vi "SystemMessageDialogBox_DynamicLaunch.vi"(6 "ErrorMessageToProcess":errorcluster, 8 "ErrorIn":errorcluster, 9 "Timeout (-1)":i32=-1, 10 "CorrAct":string, 11 "Source":string) -> (0 "ErrorOut":errorcluster)   [LabVIEW 2018]
doc: "Call this modal dialog when an error occurs. This VI logs the error to a file to aid in diagnosis.\n\nThe CorrAct (Corrective Action) input can be used to suggest a solution to the user.\n\nCopyright © 2016 Epimedia, Inc. All Rights Reserved.\n\nThe Epimedia Application Library is Copyright © 2009-2016 Epimedia, Inc. \nAll Rights Reserved. Used under license."
uses:
  Controls/SMSDataCluster.ctl
  <vilib>/Utility/sysdir.llb/System Directory Type.ctl
panel:
  in  "SMS":T1
  in  "Close":bool
  out "CorrAction":string caption="Corrective Action:"
  out "ErrorSource":string caption="Source:"
  out "ErrorCode":i32 caption="Code:"
  # "System Message"
  # "Copyright © 2016 Epimedia, Inc. All Rights Reserved.\n\nThe Epimedia Application Library is Copyright © 2009-2016 Epimedia, Inc. \nAll Rights Reserved. Used under license."
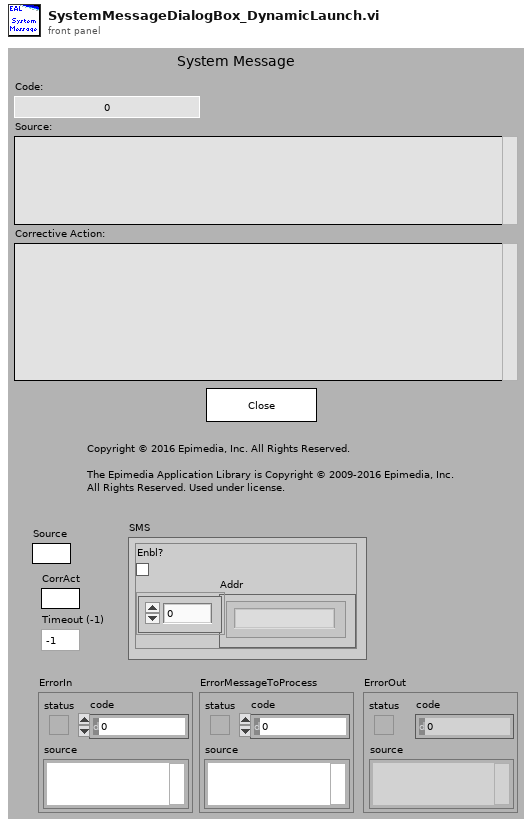
[diagram p1: front panel]
types:
  T1 = typedef "SMSDataCluster.ctl" = cluster{"Enbl?":bool, "Addr":string[]}
  T2 = enum8{"Enabled", "Disabled", "Disabled and Grayed Out"}
  T3 = typedef "System Directory Type.ctl" = i32
  T4 = enum16{"open", "replace", "create", "open or create", "replace or create", "replace or create with confirmation"}
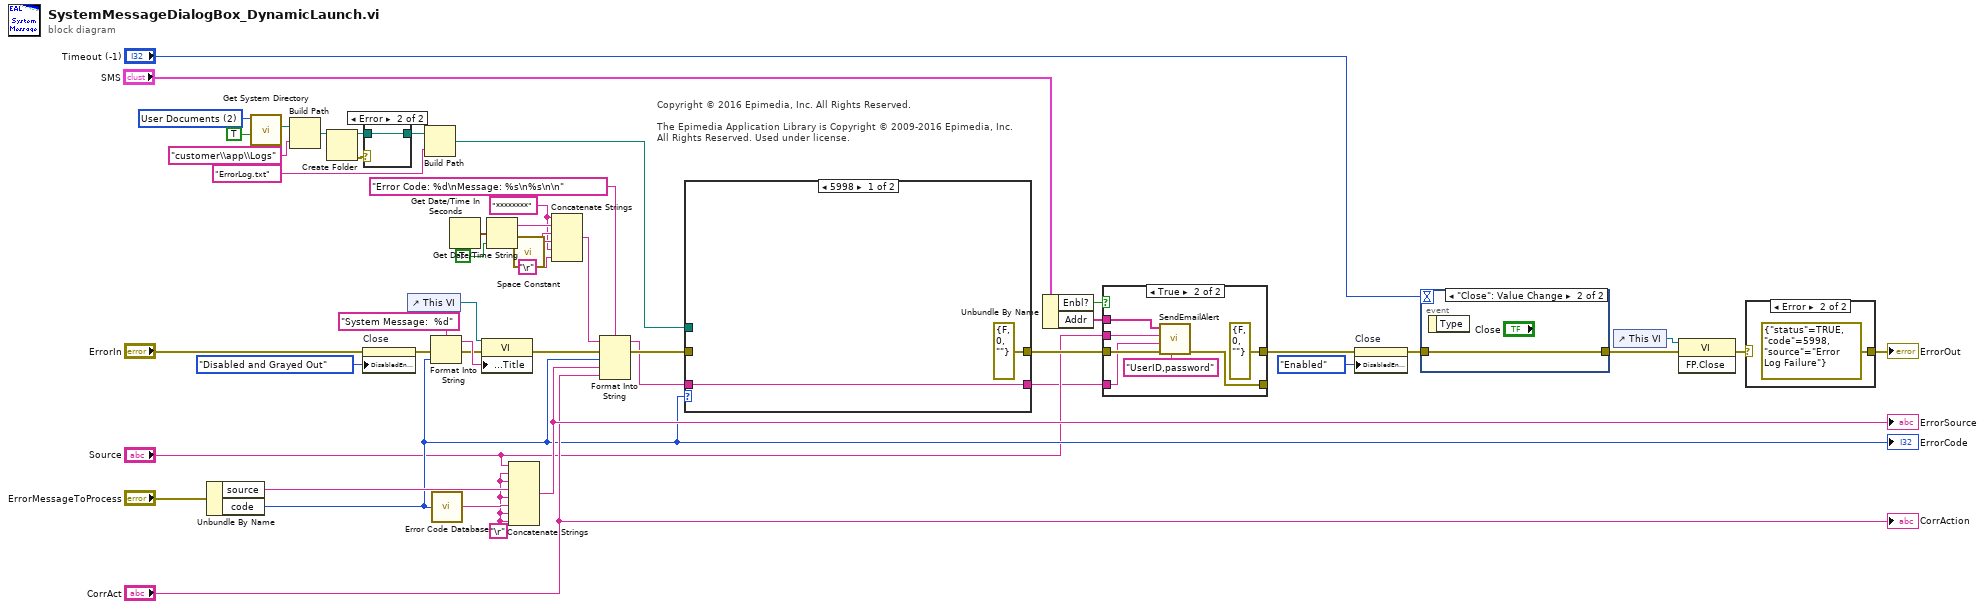
[diagram p0: block diagram]
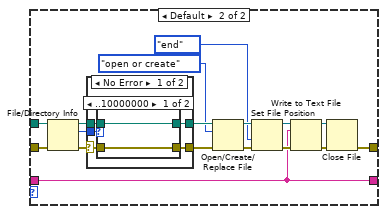
[diagram p3: hidden frame]
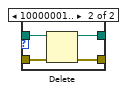
[diagram p4: hidden frame]
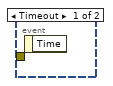
[diagram p8: hidden frame]
diagram:
  w38 = T3 2 items=["User Home"=0, "User Desktop"=1, "User Documents"=2, "User Application Data"=3, "User Preferences"=4, "User Temporary"=5, "Public Documents"=6, "Public Application Data"=7, "Public Preferences"=8, "Public Cache"=13, "System Core Libraries"=9, "System Installed Libraries"=10, "Application Files"=11, "Boot Volume Root"=12] ("system directory type")
  w41 = "********" ("string")
  w22 = "\r"
  # "Copyright © 2016 Epimedia, Inc. All Rights Reserved.\n\nThe Epimedia Application Library is Copyright © 2009-2016 Epimedia, Inc. \nAll Rights Reserved. Used under license."
  n1 = Unbundle By Name("ErrorMessageToProcess") -> ("source"=w23:string, "code"=w6:i32)
  "ErrorCode" <- w6
  n2 = call <vilib>:"Get System Directory.vi"("create directory if not found? (F)"=TRUE, "system directory type"=w38) -> ("system directory"=w37:path)  [unwired: 9 in]
  n3 = Build Path(base path=w37, name or relative path="customer\\app\\Logs") -> (appended path=w30:path)
  n4 = Create Folder(path (use dialog)=w30) -> (created path=w32:path, error out=w33:errorcluster)  [unwired: 2 in, 1 out]
  n5 = property on="Close" class="Bool"(error in="ErrorIn", "DisabledEnum"=T2."Disabled and Grayed Out" ("Disabled")) -> (error out=w20:errorcluster)  [unwired: 1 in, 1 out]
  n6 = case shown="Error" w33 {
    tunnel: w32 -> [w51 w52]
    tunnel: [w51 w52] -> w31
    frame No Error {
    }
    frame Error {
    }
  }
  n7 = control-ref of="This VI"() -> (w28:refnum<vi>)
  n8 = Build Path(base path=w31, name or relative path="ErrorLog.txt") -> (appended path=w29:path)
  n9 = Format Into String(format string="System Message:  %d" ("string"), error in=w20, w6) -> (resulting string=w26:string, error out=w25:errorcluster)  [unwired: 1 in]
  n10 = call <vilib>:"Error Code Database.vi"("Error Code"=w6) -> ("Error Text"=w42:string)
  n11 = Get Date/Time In Seconds() -> (seconds since 1Jan1904=w49:timestamp)
  n12 = property class="VI"(reference=w28, error in=w25, "Front Panel.Title"=w26) -> (error out=w24:errorcluster)  [unwired: 1 out]
  n13 = Get Date/Time String(seconds (now)=w49, want seconds? (F)=TRUE) -> (date string=w48:string, time string=w47:string)  [unwired: 1 out]
  n14 = Concatenate Strings("Source", w22, w22, w23, w22, w42, w22, w22) -> (w15:string)
  "ErrorSource" <- w15
  n15 = call <vilib>:"Space Constant.vi"() -> ("String"=w45:string)
  n16 = Concatenate Strings(w41, w48, w45, w47, w41, "\r") -> (w43:string)
  n17 = Format Into String(format string="Error Code: %d\nMessage: %s\n%s\n\n", initial string=w43, error in=w24, w6, w15, "CorrAct") -> (resulting string=w12:string, error out=w36:errorcluster)
  n18 = case shown="5998" w6 {
    tunnel: w36 -> [_ w58]
    tunnel: w29 -> [_ w57]
    tunnel: [errorcluster {"status"=FALSE, "code"=0, "source"=""} ("error out") w56] -> w7
    tunnel: w12 -> [w53 w55]
    tunnel: [w53 w55] -> w4
    frame 5998 {
    }
    frame Default {
      n19 = File/Directory Info(path=w57, error in=w58) -> (path out=w68:path, size=w70:i64, error out=w71:errorcluster)  [unwired: 4 out]
      n20 = case shown="No Error" w71 {
        selector: w71 -> [w72 _]
        tunnel: [w76 _] -> w67
        tunnel: w68 -> [w75 w83]
        tunnel: [w74 w83] -> w69
        tunnel: w70 -> [w73 _]
        frame No Error {
          n21 = case shown="..10000000" w73 {
            tunnel: w72 -> [w77 w82]
            tunnel: [w77 w81] -> w76
            tunnel: w75 -> [w78 w80]
            tunnel: [w78 w79] -> w74
            frame ..10000000 {
            }
            frame 10000001.. {
              n22 = Delete(path (use dialog)=w80, error in=w82) -> (deleted path=w79:path, error out=w81:errorcluster)  [unwired: 3 in, 1 out]
            }
          }
        }
        frame Error {
        }
      }
      n23 = Open/Create/Replace File(file path (use dialog)=w69, error in=w67, operation (0:open)=T4."open or create") -> (refnum out=w64:refnum<file>, error out=w63:errorcluster)  [unwired: 4 out]
      n24 = Set File Position(refnum=w64, from (0:start)=enum16{"start", "end", "current"}."end", error in=w63) -> (refnum out=w65:refnum<file>, error out=w66:errorcluster)  [unwired: 1 out]
      n25 = Write to Text File(file (use dialog)=w65, text=w55, error in=w66) -> (refnum out=w61:refnum<file>, error out=w60:errorcluster)  [unwired: 2 out]
      n26 = Close File(refnum=w61, error in=w60) -> (error out=w56:errorcluster)  [unwired: 1 out]
    }
  }
  n27 = Unbundle By Name("SMS") -> ("Enbl?"=w2:bool, "Addr"=w1:string[])
  n28 = case shown="True" w2 {
    tunnel: w7 -> [w84 w91]
    tunnel: [w84 errorcluster {"status"=FALSE, "code"=0, "source"=""} ("ErrorOut")] -> w8
    tunnel: [_ w89] -> _
    tunnel: "Source" -> [_ w87]
    tunnel: w4 -> [_ w86]
    tunnel: w1 -> [_ w85]
    frame False {
    }
    frame True {
      n29 = call "SendEmailAlert.vi"("UserID,PW"="UserID,password", "ErrorIn"=w91, "Body"=w86, "Subject"=w87, "RecipientsIn"=w85) -> ("ErrorOut"=w89:errorcluster)  [unwired: 6 in]
    }
  }
  n30 = property on="Close" class="Bool"(error in=w8, "DisabledEnum"=T2."Enabled" ("Disabled")) -> (error out=w17:errorcluster)  [unwired: 1 in, 1 out]
  n31 = event shown="[1] \"Close\": Value Change" {
    selector: _ -> [_ _]
    dyn-events: _ -> [_ _]
    timeout: "Timeout (-1)" -> [_ _]
    tunnel: w17 -> [_ w92]
    tunnel: [_ w92] -> w16
    event Timeout {
      n32 = event-data() -> ()  [unwired: 2 out]
    }
    event "Close": Value Change {
      n33 = event-data() -> ()  [unwired: 2 out]
    }
  }
  n34 = control-ref of="This VI"() -> (w11:refnum<vi>)
  n35 = invoke class="VI" method="FP.Close"(reference=w11, error in=w16) -> (error out=w10:errorcluster)  [unwired: 1 in, 2 out]
  n36 = case shown="Error" w10 {
    selector: w10 -> [w93 _]
    tunnel: [w93 errorcluster {"status"=TRUE, "code"=5998, "source"="Error Log Failure"} ("error IO")] -> w9
    frame No Error {
    }
    frame Error {
    }
  }
  "ErrorOut" <- w9
  "CorrAction" <- "CorrAct"
